vi "Main.vi"(11 "Module Admin":refnum<class "Delacor_lib_QMH_Module Admin.lvclass">) -> ()   [LabVIEW 2019, in "Panther Dashboard.lvlib"]
doc: "Panther Dashboard For DQMH®\n\nDeveloped and maintained by:\nPantherLAB\n\nMain Contributor- Developer:\n\n» Enrique Noé Arias\n\nBrainstorming & Code Reviews:\n\n» Matthias Baudot\n» Fabiola De La Cueva\n» Christopher Farmer\n» Cyril Gambini\n» Joerg Hampel\n» Olivier Jourdan\n» Cesar Muñoz\n» Darren Nattinger\n» Luis Orozco\n» Sam Taggart\n» Diego Torres"
uses:
  Panther Dashboard.lvlib
  <vilib>/Delacor/Delacor QMH/Libraries/Module Admin_class/Delacor_lib_QMH_Module Admin.lvclass
  refresh--button.ctl
  Module Data--cluster.ctl
  Maps List and refs--cluster.ctl
  <vilib>/National Instruments/Tree Map/Tree Map Data.ctl
  DQMH Modules Info--cluster.ctl
  Module type--enum.ctl
  Project References--cluster.ctl
  Selection Type--enum.ctl
  <vilib>/Delacor/Delacor QMH/Libraries/Module Admin_class/Delacor_lib_QMH_Module Admin.lvclass/Delacor_lib_QMH_Module Admin.ctl
  References Updated Argument--cluster.ctl
  DQMH Tools Menu--enum.ctl
  <vilib>/Delacor/Delacor QMH/Libraries/Message Queue_class/Delacor_lib_QMH_Message Queue.lvclass/Delacor_lib_QMH_Message Queue.ctl
  Expand Results Argument--cluster.ctl
  Execute Default Event Request Argument--cluster.ctl
  Tree DQMH Selection Argument--cluster.ctl
  Scan DQMH Modules Argument--cluster.ctl
  Stop Argument--cluster.ctl
  <vilib>/Utility/miscctls.llb/LVPointTypeDef.ctl
  <vilib>/Delacor/Delacor QMH/Libraries/Message Queue_class/Delacor_lib_QMH_Enqueue Message (Single).vi
  <vilib>/Delacor/Delacor QMH/Libraries/Module Admin_class/Delacor_lib_QMH_Get External Launch.vi
  <vilib>/National Instruments/Tree Map/API/List Roots.vi
  <vilib>/National Instruments/Tree Map/Utility/Into Tree Control Items.vi
  <vilib>/Platform/browser.llb/Open URL in Default Browser (string).vi
  <vilib>/Platform/browser.llb/Open URL in Default Browser (path).vi
  <vilib>/Utility/error.llb/Error Cluster From Error Code.vi
  <vilib>/ErrorRing/Error Ring.xnode
  <vilib>/Delacor/Delacor QMH/Libraries/Message Queue_class/Delacor_lib_QMH_Message Queue.lvclass
  <vilib>/National Instruments/Tree Map/Tree Map.lvlib
  <vilib>/Delacor/Delacor QMH/Libraries/Scripting API/DQMH_Scripting API.lvlib
panel:
  in  "Targets":string(combo)
  in  "Projects":string(combo)
  in  "Expanded Results":bool
  in  "Include Dependencies":bool
  in  "Scan Project":T1
  in  "Modules Tree":string(tree) caption="Tree 2"
  in  "Validate Module":bool
  in  "Edit":bool
  in  "Edit":bool
  in  "Module Description":string
  out "Event Connector Pane":picture
  in  "Event Description":string
  in  "Module ID":i32=-1 min=-1 max=1000 step=1 format="Module ID %d"
  in  "Create Module Template":bool
  in  "Create RT Tester":bool
  in  "Add Unit Test":bool
  in  "Rename Module":bool
  in  "Add Module":bool
  in  "Rename Event":bool
  in  "Convert Event":bool
  in  "Remove Event":bool
  in  "Add Event":bool
  out "Progress":u16(slide) scale=0.0..1.0
  out "Messages":string
  in  "Theme":bool=TRUE
  in  "About":bool=TRUE
  out "error out":errorcluster
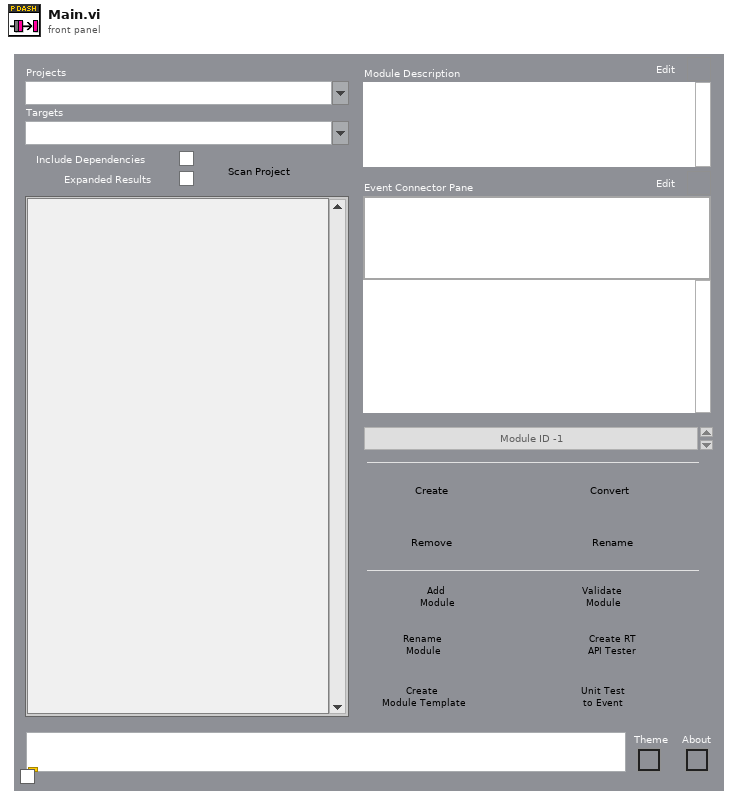
[diagram p1: front panel]
types:
  T1 = typedef "Panther Dashboard.lvlib/refresh--button.ctl" = bool
  T2 = typedef "Panther Dashboard.lvlib/Broadcast Events--cluster.ctl" = cluster{"Module Did Init":refnum<user-event>, "Status Updated":refnum<user-event>, "Error Reported":refnum<user-event>, "Module Did Stop":refnum<user-event>, "Update Module Execution Status":refnum<user-event>, "References Updated":refnum<user-event>, "Projects Updated":refnum<user-event>, "Targets Updated":refnum<user-event>}
  T3 = typedef "Panther Dashboard.lvlib/Request Events--cluster.ctl" = cluster{"Stop Module":refnum<user-event>, "Show Panel":refnum<user-event>, "Hide Panel":refnum<user-event>, "Get Module Execution Status":refnum<user-event>, "Show Diagram":refnum<user-event>, "Scan DQMH Modules":refnum<user-event>, "Tree DQMH Selection":refnum<user-event>, "Open Module API Tester":refnum<user-event>, "Execute Default Event Request":refnum<user-event>, "Expand Results":refnum<user-event>}
  T4 = typedef "Panther Dashboard.lvlib/Selection Type--enum.ctl" = enum16{"Broadcast", "Request", "Module", "Public API"}
  T5 = typedef "Panther Dashboard.lvlib/Module Data--cluster.ctl" = cluster{"Maps":T6, "DQMH Scan Results":T8, "Current Selection":cluster{"VI Ref":refnum<vi>, "DQMH Lib Ref":refnum<vi>}, "Status":string, "Module type":T9, "Module ID":i32, "Theme":bool, "Broadcast?":bool}
  T6 = typedef "Panther Dashboard.lvlib/Maps List and refs--cluster.ctl" = cluster{"Tree Map":T7, "References Map":map{string, refnum<vi>}}
  T7 = typedef "Tree Map.lvlib/Tree Map Data.ctl" = map{string, cluster{"Child Paths Set":set{string}, "Name":string, "Data":string, "Attributes":map{string, string}}}
  T8 = typedef "Panther Dashboard.lvlib/DQMH Modules Info--cluster.ctl" = cluster{"All DQMH Modules Refs":refnum<vi>[], "All Modules Descriptions":string[], "All Modules type":T9[], "Project References":T10}
  T9 = typedef "Panther Dashboard.lvlib/Module type--enum.ctl" = enum16{"Module type: Singleton", "Module type: Cloneable"}
  T10 = typedef "Panther Dashboard.lvlib/Project References--cluster.ctl" = cluster{"Project Ref":refnum<vi>, "Project Name":string, "Target":refnum<vi>, "App Ref":refnum<vi>}
  T11 = typedef "Panther Dashboard.lvlib/References Updated Argument--cluster.ctl" = cluster{"Modules":refnum<vi>[], "Modules Types":T9[], "Application Instance":refnum<vi>}
  T12 = typedef "Panther Dashboard.lvlib/DQMH Tools Menu--enum.ctl" = enum16{"Create New DQMH Event", "Remove DQMH Event", "Convert DQMH Event", "Rename DQMH Event", "Add New DQMH Module", "Create RT Tester", "Rename DQMH Module", "Validate DQMH Module", "Create DQMH Module Template", "New DQMH  Unit Test"}
  T13 = enum8{"Enabled", "Disabled", "Disabled and Grayed Out"}
  T14 = typedef "Panther Dashboard.lvlib/Expand Results Argument--cluster.ctl" = cluster{"Expand?":bool}
  T15 = typedef "Panther Dashboard.lvlib/Execute Default Event Request Argument--cluster.ctl" = cluster{"Event Name":string}
  T16 = typedef "Panther Dashboard.lvlib/Tree DQMH Selection Argument--cluster.ctl" = cluster{"Tree DQMH Sel":string}
  T17 = typedef "Panther Dashboard.lvlib/Scan DQMH Modules Argument--cluster.ctl" = cluster{"Include Dependencies":bool, "Project":string, "Target":string}
  T18 = enum32{"invalid lock state", "Not Locked", "Locked (No Password)", "Password-protected"}
  T19 = typedef "Panther Dashboard.lvlib/Stop Argument--cluster.ctl" = cluster{"Origin":string, "Exit via Stop Module Req?":bool, "Wait for Module to stop?":bool}
  T20 = typedef "LVPointTypeDef.ctl" = cluster{"Horizontal":i16, "Vertical":i16}
  T21 = enum32{"Invalid", "Standard", "Closed", "Hidden", "Minimized", "Maximized"}
  T22 = cluster{"Left Cell String":string, "Child Text":string[], "Child Tag":string, "Item Indent":i32, "Child Only?":bool, "Glyph Index":i32}[]
  T23 = typedef "Panther Dashboard.lvlib/Documentation--cluster.ctl" = cluster{"Module Description":string, "Event Description":string}
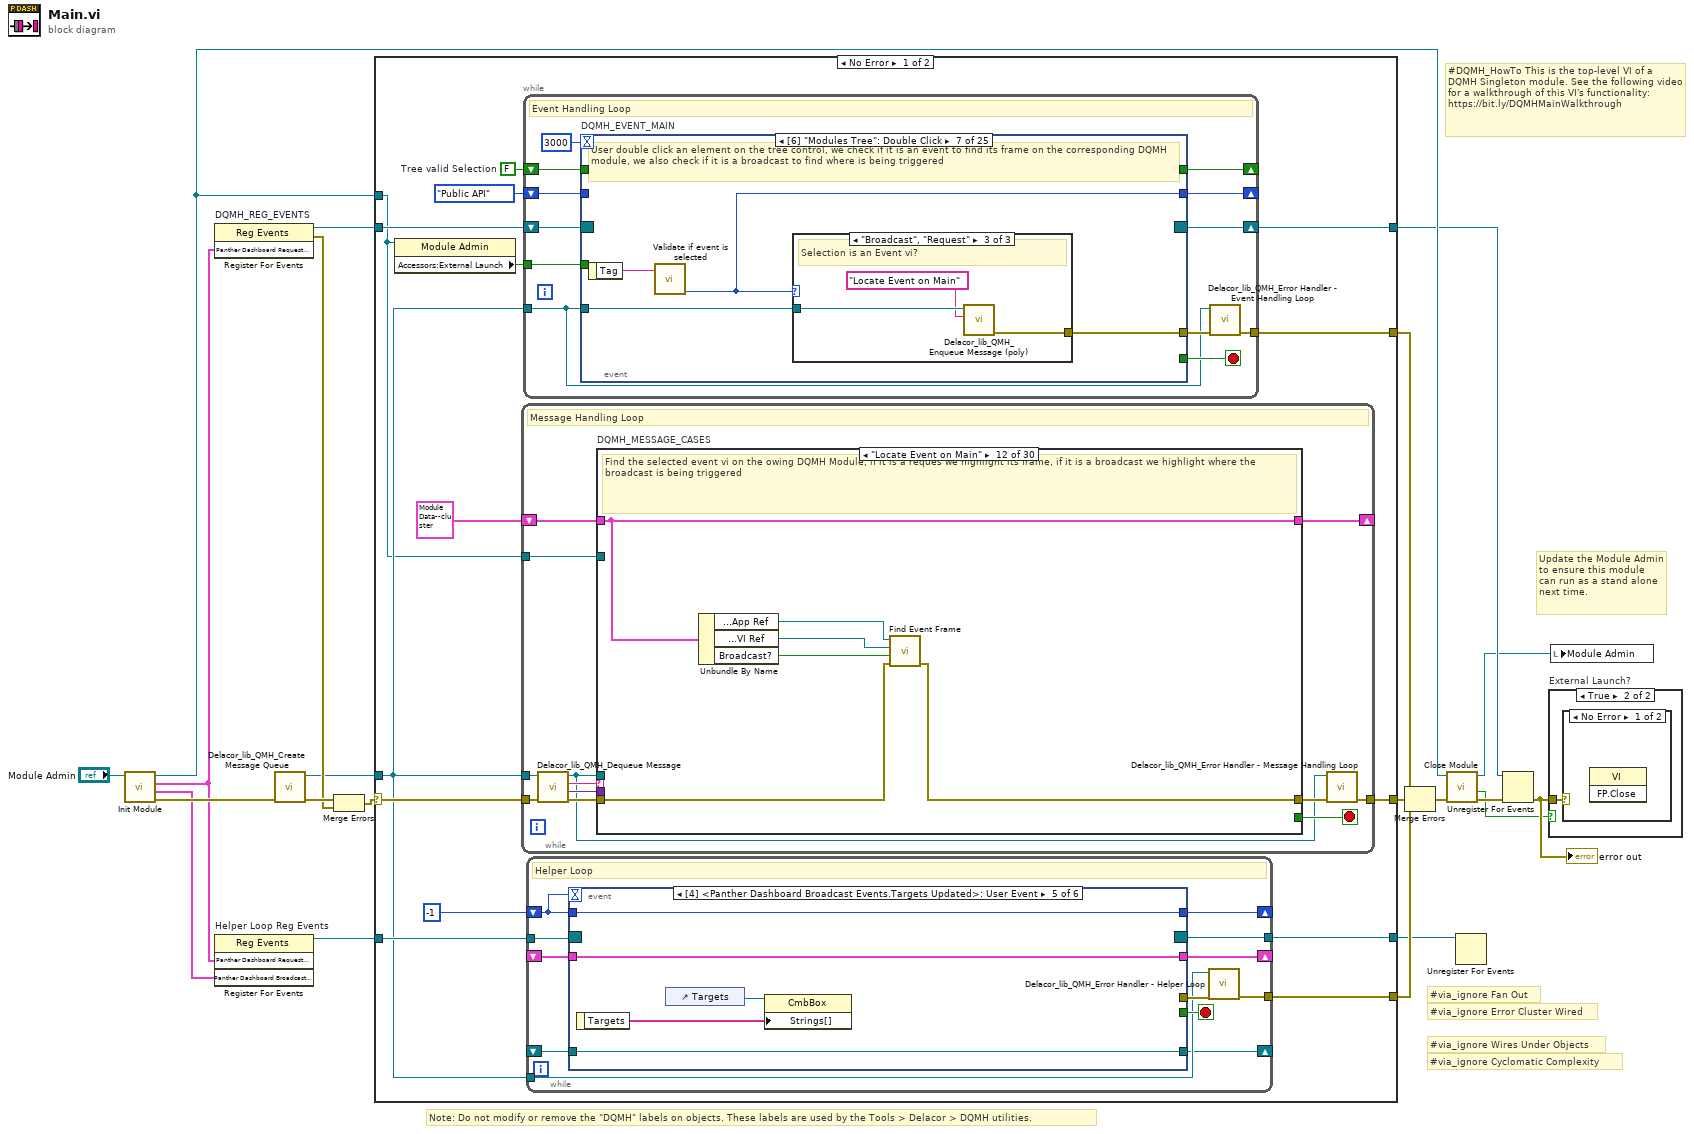
[diagram p0: block diagram]
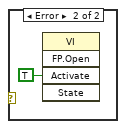
[diagram p3: hidden frame]
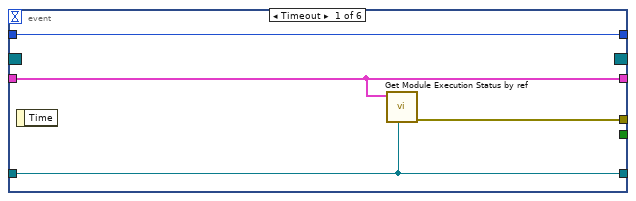
[diagram p4: hidden frame]
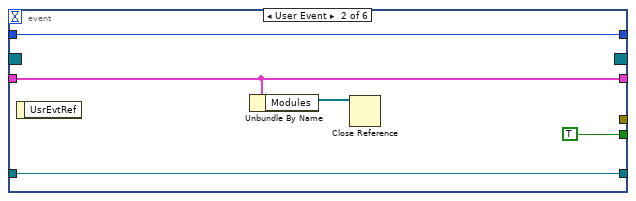
[diagram p5: hidden frame]
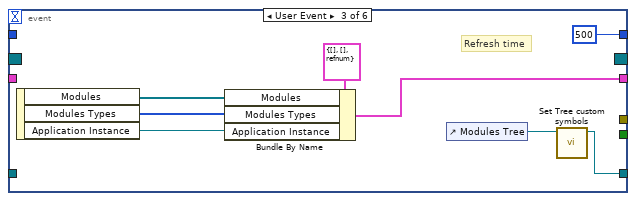
[diagram p6: hidden frame]
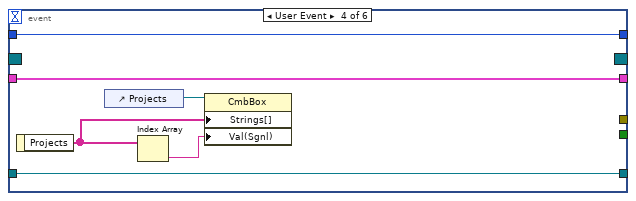
[diagram p7: hidden frame]
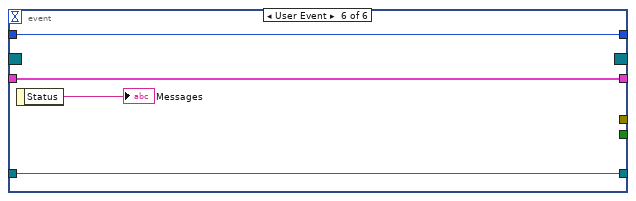
[diagram p8: hidden frame]
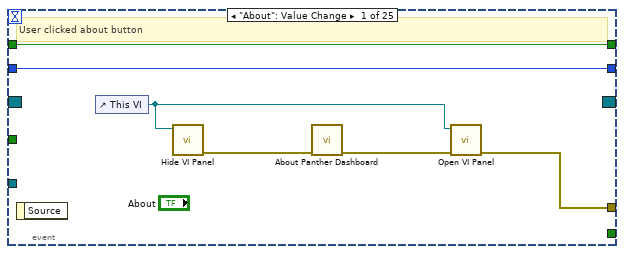
[diagram p9: hidden frame]
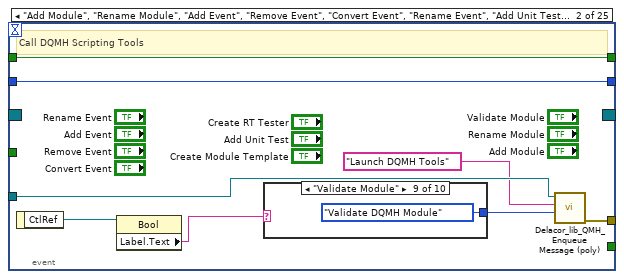
[diagram p10: hidden frame]
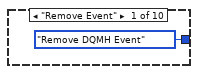
[diagram p11: hidden frame]
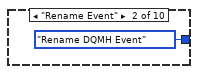
[diagram p12: hidden frame]
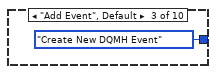
[diagram p13: hidden frame]
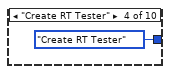
[diagram p14: hidden frame]
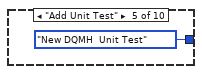
[diagram p15: hidden frame]
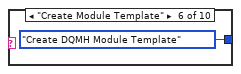
[diagram p16: hidden frame]
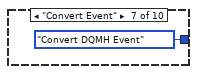
[diagram p17: hidden frame]
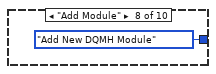
[diagram p18: hidden frame]
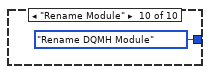
[diagram p19: hidden frame]
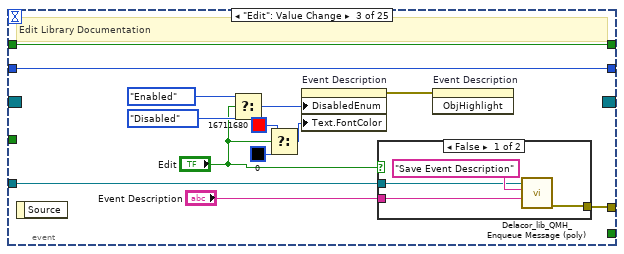
[diagram p20: hidden frame]
diagram:
  # "#via_ignore Fan Out"
  # "#via_ignore Cyclomatic Complexity"
  # "#via_ignore Wires Under Objects"
  # "#via_ignore Error Cluster Wired"
  # "#DQMH_HowTo This is the top-level VI of a DQMH Singleton module. See the following video for a walkthrough of this VI's functionality: https://bit.ly/DQMHMainWalkthrough"
  # "Note: Do not modify or remove the \"DQMH\" labels on objects. These labels are used by the Tools > Delacor > DQMH utilities."
  # "Update the Module Admin to ensure this module can run as a stand alone next time."
  n1 = call "Init Module.vi"("Singleton Module Admin in"="Module Admin") -> ("error out"=w20:errorcluster, "Panther Dashboard Broadcast Events"=w1:T2, "Panther Dashboard Request Events"=w2:T3, "Singleton Module Admin out"=w11:refnum<class "Delacor_lib_QMH_Module Admin.lvclass">)  [unwired: 7 in]
  n2 = register-events "DQMH_REG_EVENTS"(w2) -> (reference out=w9:refnum<event-registration>, error out=w13:errorcluster)  [unwired: 2 in]
  n3 = register-events "Helper Loop Reg Events"(w2, w1) -> (reference out=w4:refnum<event-registration>)  [unwired: 2 in, 1 out]
  n4 = call <vilib>:"Delacor_lib_QMH_Create Message Queue.vi"("error in"=w20) -> ("error out"=w15:errorcluster, "Message Queue"=w8:refnum<class "Delacor_lib_QMH_Message Queue.lvclass">)  [unwired: 9 in]
  n5 = Merge Errors(w15, w13) -> (w14:errorcluster)
  n6 = case shown="No Error" w14 {
    selector: w14 -> [w34 w689]
    tunnel: [w36 w688] -> w21
    tunnel: [w32 w687] -> w10
    tunnel: w9 -> [w30 w687]
    tunnel: w8 -> [w26 w682]
    tunnel: [w35 _] -> w18
    tunnel: w11 -> [w23 w683]
    tunnel: w4 -> [w29 w681]
    tunnel: [w28 w681] -> w3
    tunnel: [w33 _] -> w12
    frame No Error {
      w25 = FALSE  # Tree valid Selection
      n7 = property class="Module Admin"(reference=w23) -> ("Accessors:External Launch"=w22:bool)  [unwired: 1 in, 2 out]
      n8 = while {
        tunnel: w26 -> [w326]
        shift-right: [w330] -> _
        shift-left: T5 {"Maps"={"Tree Map"={}, "References Map"={}}, "DQMH Scan Results"={"All DQMH Modules Refs"=[], "All Modules Descriptions"=[], "All Modules type"=[], "Project References"={"Project Ref"=refnum, "Project Name"="", "Target"=refnum, "App Ref"=refnum}}, "Current Selection"={"VI Ref"=refnum, "DQMH Lib Ref"=refnum}, "Status"="", "Module type"=enum."Module type: Singleton", "Module ID"=0, "Theme"=FALSE, "Broadcast?"=FALSE} ("Data Cluster") -> [w331]
        tunnel: w34 -> [w334]
        tunnel: [w332] -> w36
        tunnel: w23 -> [w324]
        stop <- w329 stop-if-true
        # "Message Handling Loop"
        n9 = call-dynamic "Delacor_lib_QMH_Dequeue Message.vi"("error in"=w334, "Message Queue in"=w326) -> ("error out"=w333:errorcluster, "Message Data"=w327:variant, "Message"=w328:string, "Message Queue out"=w325:refnum<class "Delacor_lib_QMH_Message Queue.lvclass">)  [unwired: 6 in]
        n10 = case "DQMH_MESSAGE_CASES" shown="\"Locate Event on Main\"" w328 {
          selector: w328 -> [_ w379 _ _ _ _ _ _ _ _ _ _ _ _ _ _ w551 _ w574 _ _ _ _ _ _ _ _ _ _ w668]
          tunnel: w325 -> [w346 _ _ _ _ _ _ _ _ _ _ _ _ _ _ _ _ _ _ _ _ _ _ _ _ _ _ w638 w660 _]
          tunnel: w333 -> [w364 w382 w384 w408 w416 w423 w430 w456 w472 w477 w478 w484 w502 w518 w537 w544 w556 w569 w579 w592 w599 w606 w609 w620 w628 w633 w635 w645 w666 w670]
          tunnel: [w363 w375 w384 w407 w415 w423 w430 w455 w471 w476 w483 w489 w500 w516 w539 w543 w554 w570 w577 w584 w598 w605 w608 w620 w624 w632 w635 w641 w663 w671] -> w335
          tunnel: w331 -> [w352 w381 w383 w395 w413 w421 w429 w451 w467 w475 w482 w488 w495 w514 w541 w546 w550 w567 w573 w591 w597 w604 w611 w619 w629 w631 w634 w640 w652 w669]
          tunnel: [w351 w381 w383 w400 w413 w421 w429 w445 w467 w475 w482 w488 w495 w514 w541 w546 w548 w567 w571 w587 w595 w604 w611 w619 w629 w631 w634 w640 w652 w669] -> w330
          tunnel: [_ _ _ _ _ _ _ _ _ _ _ _ _ _ _ _ _ _ _ _ _ _ _ _ _ _ _ _ w659 _] -> w329
          tunnel: w327 -> [_ w380 _ w403 _ _ _ w454 w469 _ _ _ w498 _ _ _ w552 _ w575 w589 w596 w603 _ _ _ _ _ w639 w658 _]
          tunnel: w324 -> [w353 _ _ _ _ _ _ _ _ _ _ _ _ _ _ _ _ _ _ _ _ _ _ _ _ _ _ w637 w653 _]
          frame "Initialize" {
            w343 = "Panther Dashboard for DQMH" ("format string")
            # "#via_ignore Overlapping Controls"
            # "Scripting not\nallowed on RTE"
            # "Initialize - Any operation that needs to be done before the module can receive messages. Synchronize Caller Events.vi will inform Start Module.vi that the module has launched and is ready to receive messages. Module Did Init.vi will broadcast that the module initialized."
            n11 = call "Synchronize Caller Events.vi"("error in (no error)"=w364, "Singleton Module Admin in"=w353) -> ("error out"=w361:errorcluster, "Singleton Module Admin out"=w348:refnum<class "Delacor_lib_QMH_Module Admin.lvclass">)  [unwired: 8 in]
            n12 = invoke on="Modules Tree" class="Tree (strict)" method="Edit Tree Items.Delete"() -> ()  [unwired: 5 in, 5 out]
            n13 = property on="Property Node" class="Module Admin"(reference=w348) -> ("Accessors:External Launch"=w357:bool)  [unwired: 1 in, 2 out]
            n14 = call "Scan For App Projects.vi"("error in"=w361) -> ("error out"=w360:errorcluster)  [unwired: 10 in]
            n15 = Select(t=T21."Hidden" ("State"), s=w357, f=T21."Standard" ("State")) -> (s? t:f=w354:T21)
            n16 = property on="Event Connector Pane" class="Pict"("Origin"=T20 {"Horizontal"=-5, "Vertical"=-3}) -> ()  [unwired: 2 in, 2 out]
            n17 = call "Module Name--constant.vi"() -> ("Module Name"=w349:string)  [unwired: 11 in]
            n18 = property on="Property Node" class="VI"("Front Panel.Title"=w343, "Front Panel.IsFrontmost"=TRUE ("Front Panel Window:Is Frontmost")) -> (reference out=w359:refnum<vi>, error out=w366:errorcluster)  [unwired: 2 in]
            n19 = call "Module Did Init.vi"("error in (no error)"=w360, "Initialized?"=TRUE, "Origin"=w349) -> ("error out"=w338:errorcluster)  [unwired: 8 in]
            n20 = invoke on="Invoke Node" class="VI" method="FP.Open"(reference=w359, error in=w366, "State"=w354) -> (reference out=w358:refnum<vi>, error out=w365:errorcluster)  [unwired: 2 in, 3 out]
            n21 = call "Read Theme from Config.vi"("error in"=w338) -> ("error out"=w337:errorcluster, "Theme"=w336:bool)  [unwired: 9 in]
            n22 = property on="Modules Tree" class="Tree (strict)"("Allow Item Drag"=TRUE ("Drag/Drop:Allow Dragging"), "SelColor"=u32 8355711) -> ()  [unwired: 2 in, 2 out]
            n23 = invoke on="Invoke Node" class="VI" method="FP.Center"(reference=w358, error in=w365) -> (reference out=w344:refnum<vi>, error out=w362:errorcluster)  [unwired: 1 in, 1 out]
            n24 = Bundle By Name(cluster=w352, "Module ID"=-1, "Status"=w343) -> (w351:T5)
            n25 = local write "Messages"(w343) -> ()
            n26 = disable-structure shown="RUN_TIME_ENGINE==True" {
              disable-tunnel: w337 -> [w371 w374]
              disable-tunnel: [w370 w373] -> w363
              disable-tunnel: w346 -> [w369 _]
              disable-tunnel: w336 -> [w367 _]
              frame condition #0 (active) {
                n27 = call-poly <vilib>:"Delacor_lib_QMH_Enqueue Message (poly).vi"("error in"=w371, "Message Data"=w367, "Message"="Theme", "Message Queue in"=w369) -> ("error out"=w370:errorcluster)  [unwired: 6 in, 1 out]
              }
              frame condition #1 {
                n28 = call "Stop Module.vi"("error in"=w374, "Origin"="Self") -> ("error out"=w373:errorcluster)  [unwired: 9 in]
              }
            }
            n29 = invoke class="VI" method="Default Vals.Reinit All"(reference=w344, error in=w362) -> ()  [unwired: 1 in, 3 out]
            "Progress" <- u16 0 ("Progress")
          }
          frame "Refresh Targets" {
            # "When the User selects a Project triggers this task to scan all the targets available"
            n30 = Variant To Data(error in=w382, type=w379, Variant=w380) -> (data=w378:string, error out=w377:errorcluster)
            n31 = call "Get all Targets.vi"("error in"=w377, "Project Selection"=w378) -> ("error out"=w375:errorcluster, "Targets"=w376:string[])  [unwired: 8 in]
            n32 = call "Targets Updated.vi"("Targets"=w376) -> ()  [unwired: 10 in, 1 out]
          }
          frame "---Module Specific---" {
            # "Separator -- The following cases handle messages specific to this Module."
          }
          frame "Scan DQMH Modules" {
            # "Scan DQMH Modules in the project and fill 2 maps one with the Vi References and the another one with the list of DQMH modules on the project"
            n33 = Variant To Data(error in=w408, type=T17 {"Include Dependencies"=FALSE, "Project"="", "Target"=""} ("Scan DQMH Modules Argument"), Variant=w403) -> (data=w401:T17, error out=w386:errorcluster)
            n34 = Unbundle By Name(w401) -> ("Project"=w388:string, "Target"=w390:string, "Include Dependencies"=w391:bool)
            n35 = invoke on="Modules Tree" class="Tree (strict)" method="Edit Tree Items.Delete"(error in=w386) -> ()  [unwired: 4 in, 5 out]
            n36 = call "Close vi references.vi"("Data Cluster"=w395) -> ("error out"=w404:errorcluster)  [unwired: 10 in]
            n37 = disable-structure shown="Disabled" {
              disable-tunnel: w386 -> [w409 _]
              frame Disabled {
                n38 = call <vilib>:"Set Busy.vi"("error in (no error)"=w409) -> ()  [unwired: 9 in, 2 out]
              }
              frame Enabled {
              }
            }
            n39 = local write "Include Dependencies"(w391) -> ()
            n40 = Format Into String(format string="Panther Dashboard for DQMH: %s", w388) -> (resulting string=w392:string)  [unwired: 2 in, 1 out]
            n41 = control-ref of="Progress"() -> (w387:refnum<vi>)
            n42 = local read "Expanded Results"() -> (w394:bool)
            n43 = property on="Property Node" class="VI"("Front Panel.Title"=w392) -> ()  [unwired: 2 in, 2 out]
            n44 = call "Scan DQMH Modules and create Maps.vi"("Progress bar"=w387, "error in"=w404, "Include Dependencies"=w391, "Target Selection"=w390, "Project"=w388) -> ("error out"=w406:errorcluster, "Tree Map out"=w389:T7, "map ref out"=w396:map{string, refnum<vi>}, "DQMH Modules Info"=w399:T8)  [unwired: 3 in]
            n45 = control-ref of="Modules Tree"() -> (w397:refnum<vi>)
            n46 = Bundle By Name(cluster=w395, "DQMH Scan Results"=w399, "Maps.References Map"=w396, "Maps.Tree Map"=w389) -> (w400:T5)
            n47 = call "Expand Results.vi"("error in"=w406, "Expand?"=w394) -> ("error out"=w405:errorcluster)  [unwired: 9 in]
            n48 = call <vilib>:"Tree Map to Tree Control Items.vi"("Tree Map In"=w389) -> ("Tree Control Items"=w398:T22)  [unwired: 10 in]
            n49 = call "Draw Tree.vi"("Tree Control Items"=w398, "TreeControl in"=w397) -> ("error out"=w385:errorcluster)  [unwired: 9 in]
            n50 = Merge Errors(w386, w405) -> (w407:errorcluster)
            n51 = call <vilib>:"Unset Busy.vi"("error in (no error)"=w385) -> ()  [unwired: 10 in, 1 out]
          }
          frame "Drag VI" {
            # "This is the functionality alowing drag and drop the current selection to your code, you can build code using panther Dashboard."
            n52 = Unbundle By Name(w413) -> ("DQMH Scan Results.Project References.App Ref"=w412:refnum<vi>, "DQMH Scan Results.Project References.Target"=w411:refnum<vi>, "Current Selection.VI Ref"=w410:refnum<vi>)
            n53 = call "Drop Event into subVI.vi"("Current Selection.VI Ref"=w410, "Target"=w411, "App Ref"=w412) -> ("error out"=w414:errorcluster)  [unwired: 8 in]
            n54 = Merge Errors(w414, w416) -> (w415:errorcluster)
          }
          frame "Who is launching this module?" {
            w422 = 0  # Start Module.vi index
            # "Find all the VIS calling the Start Module.vi of the selected module library"
            n55 = Unbundle By Name(w421) -> ("Theme"=w420:bool, "DQMH Scan Results.Project References.App Ref"=w419:refnum<vi>, "DQMH Scan Results.Project References.Target"=w418:refnum<vi>, "Current Selection.DQMH Lib Ref"=w417:refnum<vi>)
            n56 = call "Find some Public API VI.vi"("Theme"=w420, "Public Api file index"=w422, "Library in"=w417, "Target"=w418, "App Ref"=w419) -> ()  [unwired: 7 in]
          }
          frame "Who is registered to this module's broadcasts?" {
            w428 = 2  # Obtain Broadcast Events for Registration.vi index
            # "Find all the VIS calling the Obtain broadcast events for registration of the selected module library"
            n57 = Unbundle By Name(w429) -> ("Theme"=w427:bool, "DQMH Scan Results.Project References.App Ref"=w426:refnum<vi>, "DQMH Scan Results.Project References.Target"=w425:refnum<vi>, "Current Selection.DQMH Lib Ref"=w424:refnum<vi>)
            n58 = call "Find some Public API VI.vi"("Theme"=w427, "Public Api file index"=w428, "Library in"=w424, "Target"=w425, "App Ref"=w426) -> ()  [unwired: 7 in]
          }
          frame "Tree DQMH Selection" {
            # "There is a new selection of the DQMH Tree list, need to search and update indicators acordanly."
            n59 = Unbundle By Name(w451) -> ("Maps.Tree Map"=w450:T7, "Maps.References Map"=w449:map{string, refnum<vi>}, "DQMH Scan Results"=w448:T8)
            n60 = Variant To Data(error in=w456, type=T16 {"Tree DQMH Sel"=""} ("Tree DQMH Selection Argument"), Variant=w454) -> (data=w452:T16, error out=w455:errorcluster)
            n61 = Unbundle By Name(w452) -> ("Tree DQMH Sel"=w442:string)
            n62 = call "Get List Information.vi"("List Selection"=w442, "DQMH Scan Info"=w448, "References Map"=w449, "Tree Map"=w450) -> ("Documentation"=w446:T23, "Clone?"=w441:bool, "Vi out"=w443:refnum<vi>, "Module type"=w440:T9, "VI Connector Pane"=→"Event Connector Pane":picture, "DQMH Lib"=w444:refnum<vi>, "Broadcast?"=w431:bool)  [unwired: 1 in]
            n63 = Unbundle By Name(w446) -> ("Module Description"=w439:string, "Event Description"=w438:string)
            n64 = control-ref of="Module Description"() -> (w437:refnum<vi>)
            n65 = control-ref of="Event Description"() -> (w436:refnum<vi>)
            n66 = control-ref of="Module ID"() -> (w432:refnum<vi>)
            n67 = Bundle By Name(cluster=w451, "Current Selection.DQMH Lib Ref"=w444, "Current Selection.VI Ref"=w443, "Module type"=w440, "Broadcast?"=w431) -> (w445:T5)
            n68 = Build Array(w439, w438) -> (w434:string[])
            n69 = Build Array(w437, w436) -> (w435:refnum<vi>[])
            n70 = call "Enable disable control.vi"("Enabled?"=w441, "Digital in"=w432) -> ()  [unwired: 10 in]
            n71 = for {
              tunnel: w435 -> [w459] mode=indexing
              tunnel: w434 -> [w458] mode=indexing
              tunnel: bool[] [FALSE, TRUE] ("Adjust Height?") -> [w457] mode=indexing
              n72 = call "Format to Bold.vi"("Adjust Height?"=w457, "String Value"=w458, "String Ref"=w459) -> ()  [unwired: 9 in]
            }
          }
          frame "Launch DQMH Tools" {
            # "Launch DQMH Tools"
            n73 = Variant To Data(error in=w472, type=DQMH_Tools_Menu--enum."Create New DQMH Event" ("DQMH Tools"), Variant=w469) -> (data=w463:T12, error out=w470:errorcluster)
            n74 = Unbundle By Name(w467) -> ("DQMH Scan Results.Project References.Project Name"=w465:string, "DQMH Scan Results.Project References.App Ref"=w466:refnum<vi>, "Current Selection.DQMH Lib Ref"=w461:refnum<vi>)
            n75 = Format Into String(format string="DQMH Tool: %s being executed ", w463) -> (resulting string=w464:string)  [unwired: 2 in, 1 out]
            n76 = call "Status Updated.vi"("Status"=w464) -> ()  [unwired: 10 in, 1 out]
            n77 = property class="Library"(reference=w461) -> ("Name"=w460:string)  [unwired: 1 in, 2 out]
            n78 = call "Launch DQMH Tools by menu.vi"("Project"=w465, "Application Instance"=w466, "error in"=w470, "Module Name"=w460, "DQMH Tools"=w463) -> ("error out"=w471:errorcluster)  [unwired: 6 in]
          }
          frame "Open Module API Tester" {
            # "Open the API Tester from the current DQMH Module Selected"
            n79 = Unbundle By Name(w475) -> ("DQMH Scan Results.Project References.App Ref"=w473:refnum<vi>, "Current Selection.DQMH Lib Ref"=w474:refnum<vi>)
            n80 = call "Open API Tester.vi"("error in"=w477, "DQMH Library Ref"=w474, "Application Instance"=w473) -> ("error out"=w476:errorcluster)  [unwired: 8 in]
          }
          frame "Find Module in project" {
            # "Find the selected module in project explorer"
            n81 = Unbundle By Name(w482) -> ("Current Selection.DQMH Lib Ref"=w481:refnum<vi>, "DQMH Scan Results.Project References.Project Ref"=w480:refnum<vi>, "DQMH Scan Results.All DQMH Modules Refs"=w479:refnum<vi>[])
            n82 = call "Find Library in Project.vi"("error in (no error)"=w478, "DQMH Modules Refs"=w479, "Project Ref"=w480, "DQMH Lib Ref"=w481) -> ("error out"=w483:errorcluster)  [unwired: 7 in]
          }
          frame "Locate Event on Main" {
            # "Find the selected event vi on the owing DQMH Module, if it is a reques we highlight its frame, if it is a broadcast we highlight where the broadcast is being triggered"
            n83 = Unbundle By Name(w488) -> ("DQMH Scan Results.Project References.App Ref"=w486:refnum<vi>, "Current Selection.VI Ref"=w487:refnum<vi>, "Broadcast?"=w485:bool)
            n84 = call "Find Event Frame.vi"("error in"=w484, "Broadcast?"=w485, "VI in"=w487, "Application Instance"=w486) -> ("error out"=w489:errorcluster)  [unwired: 7 in]
          }
          frame "Execute Default Event Request" {
            # "Execute Default Event"
            n85 = Variant To Data(error in=w502, type=T15 {"Event Name"=""} ("Execute Default Event Request Argument"), Variant=w498) -> (data=w496:T15, error out=w501:errorcluster)
            n86 = Unbundle By Name(w495) -> ("DQMH Scan Results.Project References.App Ref"=w494:refnum<vi>, "Current Selection.DQMH Lib Ref"=w493:refnum<vi>, "Module ID"=w491:i32, "Module type"=w490:T9)
            n87 = Unbundle By Name(w496) -> ("Event Name"=w492:string)
            n88 = call "Execute Default event.vi"("Module type"=w490, "Module ID"=w491, "Event"=w492, "DQMH Library Ref"=w493, "application Instance"=w494) -> ("error out"=w499:errorcluster)  [unwired: 6 in]
            n89 = Merge Errors(w501, w499) -> (w500:errorcluster)
          }
          frame "Search for Event Callers / listeners" {
            # "Invalid Ref"
            # "Search for this event callers"
            n90 = Unbundle By Name(w514) -> ("Broadcast?"=w506:bool, "Theme"=w512:bool, "DQMH Scan Results.Project References.Project Ref"=w504:refnum<vi>, "Current Selection.VI Ref"=w511:refnum<vi>)
            n91 = Select(t="Searching code registered to current broadcast selection" ("Status"), s=w506, f="Searching for Event Callers" ("Status")) -> (s? t:f=w507:string)
            n92 = call "Status Updated.vi"("error in (no error)"=w518, "Status"=w507) -> ("error out"=w517:errorcluster)  [unwired: 9 in]
            n93 = case shown="False" w506 {
              tunnel: w517 -> [w523 w530]
              tunnel: [w522 w529] -> w503
              tunnel: w511 -> [w521 w526]
              tunnel: [w520 w528] -> w510
              tunnel: w504 -> [w519 w527]
              frame False {
                # "Requests"
                n94 = call <vilib>:"Get Callers of Request VI in Project.vi"("error in"=w523, "Request VI"=w521, "Project"=w519) -> ("error out"=w522:errorcluster, "Request VI Callers"=w520:refnum<vi>[])  [unwired: 7 in]
              }
              frame True {
                # "Broadcast"
                n95 = Two Button Dialog(message="This is an exhaustive task that can take up to minutes, do you wish to continue?") -> (T button?=w525:bool)  [unwired: 2 in]
                n96 = case shown="True" w525 {
                  tunnel: w530 -> [w531 w536]
                  tunnel: [w531 w535] -> w529
                  tunnel: [_ w534] -> w528
                  tunnel: w527 -> [_ w533]
                  tunnel: w526 -> [_ w532]
                  frame False {
                  }
                  frame True {
                    n97 = call <vilib>:"Get VIs Registered for Broadcast in Project.vi"("error in"=w536, "Broadcast VI"=w532, "Project"=w533) -> ("error out"=w535:errorcluster, "VIs Registered for Broadcast"=w534:refnum<vi>[])  [unwired: 7 in]
                  }
                }
              }
            }
            n98 = call <vilib>:"Set Busy.vi"("error in (no error)"=w517) -> ()  [unwired: 9 in, 2 out]
            n99 = call <vilib>:"Clear Errors.vi"("error in (no error)"=w503, "specific error code to clear (0: all)"=5000) -> ("error out"=w515:errorcluster)  [unwired: 4 in, 1 out]
            n100 = call <vilib>:"Unset Busy.vi"("error in (no error)"=w503) -> ()  [unwired: 10 in, 1 out]
            n101 = call "Start Call to results window.vi"("Find Broadcast?"=w506, "Request VI Callers"=w510, "Event"=w511, "Theme"=w512) -> ()  [unwired: 8 in]
            n102 = call <vilib>:"Clear Errors.vi"("error in (no error)"=w515, "specific error code to clear (0: all)"=1026) -> ("error out"=w516:errorcluster)  [unwired: 4 in, 1 out]
          }
          frame "Open VI on Disk" {
            # "Open current event selection on the file system"
            n103 = Unbundle By Name(w541) -> ("Current Selection.VI Ref"=w540:refnum<vi>)
            n104 = property class="VI"(reference=w540) -> ("Path"=w538:path)  [unwired: 1 in, 2 out]
            n105 = call "Open File on Disk.vi"("error in"=w537, "file or directory path"=w538) -> ("error out"=w539:errorcluster)  [unwired: 9 in]
          }
          frame "Open File Library on Disk" {
            # "Open current Module Library selection on the file system"
            n106 = Unbundle By Name(w546) -> ("Current Selection.DQMH Lib Ref"=w545:refnum<vi>)
            n107 = property class="Library"(reference=w545) -> ("Path"=w542:path)  [unwired: 1 in, 2 out]
            n108 = call "Open File on Disk.vi"("error in"=w544, "file or directory path"=w542) -> ("error out"=w543:errorcluster)  [unwired: 9 in]
          }
          frame "Save Library Documentation" {
            # "Save the Library documentation"
            n109 = Variant To Data(error in=w556, type=w551, Variant=w552) -> (data=w549:string, error out=w555:errorcluster)
            n110 = in-place {
              in-place-border: w549 -> [w561]
              in-place-border: [w563] -> w553
              n111 = in-place-cluster #1(w550) -> ("Current Selection.DQMH Lib Ref"=w562:refnum<vi>, "DQMH Scan Results"=w559:T8)
              n112 = call "Save Library Documentation.vi"("New Description"=w561, "DQMH Modules Info In"=w559, "Library in"=w562) -> ("error out"=w563:errorcluster, "DQMH Modules Info Out"=w560:T8, "Lib out"=w558:refnum<vi>)  [unwired: 6 in]
              n113 = property class="Library"(reference=w558) -> ("Description"=w557:string)  [unwired: 1 in, 2 out]
              n114 = local write "Module Description"(w557) -> ()
              n115 = in-place-cluster #1("Current Selection.DQMH Lib Ref"=w558, "DQMH Scan Results"=w560) -> (w548:T5)
            }
            n116 = property on="Module Description" class="Str"("Text.FontColor"=u32 0) -> ()  [unwired: 2 in, 2 out]
            n117 = Merge Errors(w555, w553) -> (w554:errorcluster)
          }
          frame "Edit library Documentation" {
            # "Edit Library Documentation"
            n118 = Unbundle By Name(w567) -> ("Current Selection.DQMH Lib Ref"=w566:refnum<vi>)
            n119 = call "Get library description.vi"("Library in"=w566) -> ("error out"=w568:errorcluster, "Description"=w565:string)  [unwired: 9 in]
            n120 = local write "Module Description"(w565) -> ()
            n121 = property on="Module Description" class="Str"("Text.FontColor"=u32 16711680) -> ()  [unwired: 2 in, 2 out]
            n122 = Merge Errors(w569, w568) -> (w570:errorcluster)
          }
          frame "Save Event Description" {
            # "Save Event Description"
            n123 = Variant To Data(error in=w579, type=w574, Variant=w575) -> (data=w572:string, error out=w578:errorcluster)
            n124 = in-place {
              in-place-border: w572 -> [w582]
              in-place-border: [w583] -> w576
              n125 = in-place-cluster #2(w573) -> ("Current Selection.VI Ref"=w581:refnum<vi>)
              n126 = call "Save Event Description.vi"("Event Description"=w582, "Event Ref in"=w581) -> ("error out"=w583:errorcluster, "Event Ref out"=w580:refnum<vi>)  [unwired: 8 in]
              n127 = in-place-cluster #2("Current Selection.VI Ref"=w580) -> (w571:T5)
            }
            n128 = Merge Errors(w578, w576) -> (w577:errorcluster)
          }
          frame "Theme" {
            # "Switch to Dark or light Theme modue"
            n129 = Variant To Data(error in=w592, type=TRUE, Variant=w589) -> (data=w586:bool, error out=w585:errorcluster)
            n130 = control-ref of="This VI"() -> (w590:refnum<vi>)
            n131 = Bundle By Name(cluster=w591, "Theme"=w586) -> (w587:T5)
            n132 = call "Set Theme.vi"("Dark?"=w586, "VI in"=w590) -> ()  [unwired: 10 in]
            n133 = call "Save Theme in config.vi"("error in"=w585, "Theme"=w586) -> ("error out"=w584:errorcluster)  [unwired: 9 in]
          }
          frame "Module ID Update" {
            # "Module ID Control has value change"
            n134 = Variant To Data(error in=w599, type=0 ("Module ID"), Variant=w596) -> (data=w594:i32, error out=w598:errorcluster)
            n135 = Bundle By Name(cluster=w597, "Module ID"=w594) -> (w595:T5)
          }
          frame "Expand or Close" {
            # "Expand or Close DQMH Tree control"
            n136 = Variant To Data(error in=w606, type=T14 {"Expand?"=FALSE} ("Expand or Close Argument"), Variant=w603) -> (data=w601:T14, error out=w605:errorcluster)
            n137 = Unbundle By Name(w601) -> ("Expand?"=w600:bool)
            n138 = invoke on="Modules Tree" class="Tree (strict)" method="Open/Close.Open/Close All"("Open"=w600) -> ()  [unwired: 3 in, 4 out]
          }
          frame "Open Project Folder" {
            n139 = Unbundle By Name(w611) -> ("DQMH Scan Results.Project References.Project Ref"=w610:refnum<vi>)
            n140 = property class="Project"(reference=w610) -> ("Path"=w607:path)  [unwired: 1 in, 2 out]
            n141 = call <vilib>:"Show in File System.vi"("error in (no error)"=w609, "file or directory path"=w607) -> ("error out"=w608:errorcluster)  [unwired: 9 in]
          }
          frame "Open Antidoc Output" {
            # "When there is antidoc output"
            n142 = Unbundle By Name(w619) -> ("DQMH Scan Results.Project References.Project Ref"=w618:refnum<vi>)
            n143 = property class="Project"(reference=w618) -> ("Path"=w617:path)  [unwired: 1 in, 2 out]
            n144 = Strip Path(path=w617) -> (stripped path=w616:path)  [unwired: 1 out]
            n145 = Build Path(base path=w616, name or relative path=path "Antidoc-Output/Project-Documentation.adoc") -> (appended path=w615:path)
            n146 = call <vilib>:"Check if File or Folder Exists.vi"("path"=w615) -> ("file or folder exists?"=w613:bool, "dup path"=w614:path)  [unwired: 8 in, 1 out]
            n147 = case shown="False" w613 {
              tunnel: w614 -> [_ w623]
              frame False {
                n148 = call "Status Updated.vi"("Status"="No Antidoc Output has been found") -> ()  [unwired: 10 in, 1 out]
                n149 = call-poly <vilib>:"Open URL in Default Browser.vi"("URL"="https://www.vipm.io/package/wovalab_lib_antidoc/?utm_source=vipm_desktop") -> ()  [unwired: 5 in, 2 out]
              }
              frame True {
                n150 = call-poly <vilib>:"Open URL in Default Browser.vi"("path"=w623) -> ()  [unwired: 5 in, 2 out]
              }
            }
          }
          frame "Edit Project Description" {
            n151 = Unbundle By Name(w629) -> ("DQMH Scan Results.Project References.Project Ref"=w630:refnum<vi>, "Theme"=w627:bool)
            n152 = call "Hide Panel.vi"("error in (no error)"=w628) -> ("error out"=w626:errorcluster)  [unwired: 10 in]
            n153 = call "Project documentation.vi"("error in"=w626, "Theme"=w627, "Project in"=w630) -> ("error out"=w625:errorcluster)  [unwired: 8 in]
            n154 = call "Show Panel.vi"("error in (no error)"=w625) -> ("error out"=w624:errorcluster)  [unwired: 10 in]
          }
          frame "---Copy This Frame---" {
            # "Duplicate this frame when creating new messages.  Change this comment in the duplicated frame to describe this message."
            n155 = Merge Errors(w633) -> (w632:errorcluster)
          }
          frame "---Exit and Error Handling---" {
            # "Separator - The following cases handle errors and exit messages."
          }
          frame "Error" {
            # "Error - Check the error message data and respond accordingly. This message is sent by the \"Error Handler\" VIs at the end of each loop in this application."
            n156 = property on="Property Node" class="Module Admin"(reference=w637) -> ("Accessors:External Launch"=w636:bool)  [unwired: 1 in, 2 out]
            n157 = Variant To Data(error in=w645, type=errorcluster {"status"=FALSE, "code"=0, "source"=""} ("error constant"), Variant=w639) -> (data=w646:errorcluster, error out=w643:errorcluster)
            n158 = call "Error Reported.vi"("Error"=w646) -> ()  [unwired: 10 in, 1 out]
            n159 = case shown="True" w636 {
              tunnel: [w651 _] -> w642
              tunnel: w638 -> [w649 _]
              tunnel: w646 -> [w650 _]
              frame False {
                # "If the module is running standalone, then pop up an error dialog and call the \"Exit\" message."
                n160 = call <vilib>:"Simple Error Handler.vi"("error in (no error)"=w650) -> ()  [unwired: 4 in, 5 out]
                n161 = call-poly <vilib>:"Delacor_lib_QMH_Enqueue Message (poly).vi"("Priority Message? (F)"=TRUE, "Message"="Exit", "Message Queue in"=w649) -> ("error out"=w651:errorcluster)  [unwired: 7 in, 1 out]
              }
              frame True {
                # "If the module was launched externally, calling the Error Reported broadcast VI is the only action performed by the \"Error\" message. The module's caller can then process the error appropriately."
              }
            }
            n162 = Merge Errors(w643, w642) -> (w641:errorcluster)
            n163 = local write "error out"(w641) -> ()
          }
          frame "Exit" {
            w657 = 91  # 91: not all Exit messages will have an argument
            w659 = TRUE  # Stop the VI
            # "Release the message queue reference"
            # "Exit - Exit the application."
            n164 = Variant To Data(error in=w666, type=T19 {"Origin"="", "Exit via Stop Module Req?"=FALSE, "Wait for Module to stop?"=FALSE} ("Stop Argument"), Variant=w658) -> (data=w655:T19, error out=w662:errorcluster)
            n165 = call <vilib>:"Clear Errors.vi"("error in (no error)"=w662, "specific error code to clear (0: all)"=w657) -> ("error out"=w665:errorcluster)  [unwired: 4 in, 1 out]
            n166 = control-ref of="This VI"() -> (w654:refnum<vi>)
            n167 = invoke on="Modules Tree" class="Tree (strict)" method="Edit Tree Items.Delete"() -> ()  [unwired: 5 in, 5 out]
            n168 = call-dynamic "Delacor_lib_QMH_Release Message Queue.vi"("error in"=w665, "Message Queue"=w660) -> ("error out"=w664:errorcluster)  [unwired: 9 in]
            n169 = call "Handle Exit.vi"("Stop Argument"=w655, "Admin in"=w653, "VI reference"=w654) -> ("error out"=w661:errorcluster)  [unwired: 7 in, 1 out]
            n170 = call "Close vi references.vi"("Data Cluster"=w652) -> ()  [unwired: 10 in, 1 out]
            n171 = Merge Errors(w664, w661) -> (w663:errorcluster)
          }
          frame Default {
            # "'Default' case only runs if there is a message that isn't defined in any of the other cases.  Output a programming error."
            n172 = call "Module Name--constant.vi"() -> ("Module Name"=w667:string)  [unwired: 11 in]
            n173 = xnode ("Error Ring")("parameter 0"=w668, "parameter 1"=w667) -> ("error out"=w672:errorcluster)
            n174 = Merge Errors(w670, w672) -> (w671:errorcluster)
          }
        }
        n175 = call-dynamic "Delacor_lib_QMH_Error Handler - Message Handling Loop.vi"("error in"=w335, "Message Queue in"=w325) -> ("dup error in"=w332:errorcluster)  [unwired: 8 in, 1 out]
      }
      n176 = while {
        tunnel: w26 -> [w87]
        shift-right: [w89] -> w32
        shift-left: w30 -> [w90]
        tunnel: [w91] -> w35
        shift-right: [w85] -> _
        shift-left: w25 -> [w84]
        shift-right: [w83] -> _
        shift-left: Selection_Type--enum."Public API" ("Selection type") -> [w82]
        tunnel: w22 -> [w81]
        stop <- w88 stop-if-true
        # "Event Handling Loop"
        n177 = event "DQMH_EVENT_MAIN" shown="[6] \"Modules Tree\": Double Click" {
          selector: w90 -> [_ _ _ _ _ _ _ _ _ _ _ _ _ _ _ _ _ _ _ _ _ _ _ _ _]
          dyn-events: [_ _ _ _ _ _ _ _ _ _ _ _ _ _ _ _ _ _ _ _ _ _ _ _ _] -> w89
          timeout: 3000 -> [_ _ _ _ _ _ _ _ _ _ _ _ _ _ _ _ _ _ _ _ _ _ _ _ _]
          tunnel: [_ _ _ _ _ _ _ _ _ _ _ _ _ _ _ _ _ _ _ _ _ _ TRUE ("Discard?") _ _] -> w88
          tunnel: w87 -> [_ w105 w123 w140 w153 w159 w164 w176 w181 w206 _ w215 _ w229 w237 w245 _ _ w262 w271 _ _ w309 w318 _]
          tunnel: [w93 w106 w129 w146 w154 w160 w165 w177 w182 w207 w212 w216 w219 w230 w238 w246 w250 _ w263 w272 _ _ w312 w320 w323] -> w92
          tunnel: [w98 w100 w118 w139 w148 w156 w162 w173 w179 w202 w208 w218 w227 w232 w234 w240 w248 w252 w256 w269 w284 w297 w301 w315 w322] -> w85
          tunnel: w84 -> [w98 w100 w118 w139 w148 w156 w162 w173 w179 _ w208 w218 w227 w232 w234 w240 w248 w252 w256 w269 w284 w297 w301 w315 w322]
          tunnel: [w97 w99 w117 w134 w147 w155 w161 w172 w178 w200 w210 w217 w226 w231 w233 w239 w247 w251 w255 w268 w283 w296 w300 w314 w321] -> w83
          tunnel: w82 -> [w97 w99 w117 w134 w147 w155 _ w172 w178 _ w210 w217 w226 w231 w233 w239 w247 w251 w255 w268 w283 w296 w300 w314 w321]
          tunnel: w81 -> [_ _ _ _ _ _ _ _ _ _ _ _ _ _ _ _ _ _ _ _ w282 w295 _ _ _]
          event "About": Value Change {
            # "User clicked about button"
            n178 = event-data() -> ()  [unwired: 1 in, 1 out]
            n179 = control-ref of="This VI"() -> (w94:refnum<vi>)
            n180 = call "Hide VI Panel.vi"("VI"=w94) -> ("error out"=w96:errorcluster)  [unwired: 10 in]
            n181 = call "About Panther Dashboard.vi"("error in"=w96) -> ("error out"=w95:errorcluster)  [unwired: 10 in]
            n182 = call "Open VI Panel.vi"("error in (no error)"=w95, "VI"=w94) -> ("error out"=w93:errorcluster)  [unwired: 9 in]
          }
          event "Add Module", "Rename Module", "Add Event", "Remove Event", "Convert Event", "Rename Event", "Add Unit Test", "Create RT Tester", "Create Module Template", "Validate Module": Value Change {
            # "Call DQMH Scripting Tools"
            n183 = event-data() -> ("CtlRef"=w102:refnum<vi>)  [unwired: 1 in]
            n184 = property on="Property Node" class="Bool"(reference=w102) -> ("Label.Text"=w101:string)  [unwired: 1 in, 2 out]
            n185 = case shown="\"Validate Module\"" w101 {
              tunnel: [DQMH_Tools_Menu--enum."Remove DQMH Event" ("DQMH Tools") DQMH_Tools_Menu--enum."Rename DQMH Event" ("DQMH Tools") DQMH_Tools_Menu--enum."Create New DQMH Event" ("DQMH Tools") DQMH_Tools_Menu--enum."Create RT Tester" ("DQMH Tools") DQMH_Tools_Menu--enum."New DQMH  Unit Test" ("DQMH Tools") DQMH_Tools_Menu--enum."Create DQMH Module Template" ("DQMH Tools") DQMH_Tools_Menu--enum."Convert DQMH Event" ("DQMH Tools") DQMH_Tools_Menu--enum."Add New DQMH Module" ("DQMH Tools") DQMH_Tools_Menu--enum."Validate DQMH Module" ("DQMH Tools") DQMH_Tools_Menu--enum."Rename DQMH Module" ("DQMH Tools")] -> w103
              frame "Remove Event" {
              }
              frame "Rename Event" {
              }
              frame "Add Event", Default {
              }
              frame "Create RT Tester" {
              }
              frame "Add Unit Test" {
              }
              frame "Create Module Template" {
              }
              frame "Convert Event" {
              }
              frame "Add Module" {
              }
              frame "Validate Module" {
              }
              frame "Rename Module" {
              }
            }
            n186 = call-poly <vilib>:"Delacor_lib_QMH_Enqueue Message (poly).vi"("Message Data"=w103, "Message"="Launch DQMH Tools", "Message Queue in"=w105) -> ("error out"=w106:errorcluster)  [unwired: 7 in, 1 out]
          }
          event "Edit": Value Change {
            # "Edit Library Documentation"
            n187 = event-data() -> ()  [unwired: 1 in, 1 out]
            n188 = Select(t=T13."Enabled" ("Disabled"), s="Edit", f=T13."Disabled") -> (s? t:f=w125:T13)
            n189 = Select(t=u32 16711680, s="Edit", f=u32 0) -> (s? t:f=w120:u32)
            n190 = property on="Event Description" class="Str"("DisabledEnum"=w125, "Text.FontColor"=w120) -> (error out=w128:errorcluster)  [unwired: 2 in, 1 out]
            n191 = case shown="False" "Edit" {
              tunnel: "Event Description" -> [w132 _]
              tunnel: w123 -> [w130 _]
              tunnel: [w133 _] -> w129
              frame False {
                n192 = call-poly <vilib>:"Delacor_lib_QMH_Enqueue Message (poly).vi"("Message Data"=w132, "Message"="Save Event Description", "Message Queue in"=w130) -> ("error out"=w133:errorcluster)  [unwired: 7 in, 1 out]
              }
              frame True {
              }
            }
            n193 = invoke on="Event Description" class="Str" method="ObjHighlight"(error in=w128) -> ()  [unwired: 2 in, 3 out]
          }
          event "Edit": Value Change {
            # "#via_ignore Duplicate Control Labels"
            # "Edit Library Documentation"
            n194 = event-data() -> ()  [unwired: 1 in, 1 out]
            n195 = Select(t=T13."Enabled" ("Disabled"), s="Edit", f=T13."Disabled") -> (s? t:f=w143:T13)
            n196 = property on="Module Description" class="Str"("DisabledEnum"=w143) -> (error out=w145:errorcluster)  [unwired: 2 in, 1 out]
            n197 = invoke on="Module Description" class="Str" method="ObjHighlight"(error in=w145) -> ()  [unwired: 2 in, 3 out]
            n198 = Select(t="Edit library Documentation", s="Edit", f="Save Library Documentation") -> (s? t:f=w136:string)
            n199 = call-poly <vilib>:"Delacor_lib_QMH_Enqueue Message (poly).vi"("Message Data"="Module Description", "Message"=w136, "Message Queue in"=w140) -> ("error out"=w146:errorcluster)  [unwired: 7 in, 1 out]
          }
          event "Expanded Results": Value Change {
            # "Another Module called the \"Expand or Close\" API Method."
            n200 = event-data() -> ()  [unwired: 1 in, 1 out]
            n201 = Bundle(cluster=T14 {"Expand?"=FALSE} ("Expand or Close Argument"), "Expand?"="Expanded Results") -> (w150:T14)
            n202 = call-poly <vilib>:"Delacor_lib_QMH_Enqueue Message (poly).vi"("Message Data"=w150, "Message"="Expand or Close", "Message Queue in"=w153) -> ("error out"=w154:errorcluster)  [unwired: 7 in, 1 out]
          }
          event "Module ID": Value Change {
            # "#via_ignore Unwired Event Nodes"
            # "Module ID has value change"
            n203 = event-data() -> ()  [unwired: 1 in, 1 out]
            n204 = call-poly <vilib>:"Delacor_lib_QMH_Enqueue Message (poly).vi"("Message Data"="Module ID", "Message"="Module ID Update", "Message Queue in"=w159) -> ("error out"=w160:errorcluster)  [unwired: 7 in, 1 out]
          }
          event "Modules Tree": Double Click {
            # "User double click an element on the tree control, we check if it is an event to find its frame on the corresponding DQMH module, we also check if it is a broadcast to find where is being triggered"
            n205 = event-data() -> ("Tag"=w163:string)  [unwired: 1 in]
            n206 = call "Validate if event is selected.vi"("Tree Selection"=w163) -> ("Selection type"=w161:T4)  [unwired: 10 in]
            n207 = case shown="\"Broadcast\", \"Request\"" w161 {
              tunnel: [w168 _ w171] -> w165
              tunnel: w164 -> [w167 _ w170]
              frame "Module" {
                # "Selection is a module"
                n208 = call-poly <vilib>:"Delacor_lib_QMH_Enqueue Message (poly).vi"("Message"="Find Module in project", "Message Queue in"=w167) -> ("error out"=w168:errorcluster)  [unwired: 8 in, 1 out]
              }
              frame "Public API" {
              }
              frame "Broadcast", "Request" {
                # "Selection is an Event vi?"
                n209 = call-poly <vilib>:"Delacor_lib_QMH_Enqueue Message (poly).vi"("Message"="Locate Event on Main", "Message Queue in"=w170) -> ("error out"=w171:errorcluster)  [unwired: 8 in, 1 out]
              }
            }
          }
          event "Modules Tree": Drag Starting? {
            n210 = event-data() -> ()  [unwired: 1 in, 1 out]
            n211 = call-poly <vilib>:"Delacor_lib_QMH_Enqueue Message (poly).vi"("Message"="Drag VI", "Message Queue in"=w176) -> ("error out"=w177:errorcluster)  [unwired: 8 in, 1 out]
            n212 = event-data("Discard?"=TRUE) -> ()  [unwired: 1 in, 1 out]
          }
          event "Modules Tree": Shortcut Menu Selection (User) {
            # "User selects something from the Right Click Shortcut Menu"
            n213 = event-data() -> ("ItemTag"=w180:string)  [unwired: 1 in]
            n214 = case shown="\"Open File Library on Disk\", \"Open VI on Disk\", \"Who is launching this module?\"" w180 {
              selector: w180 -> [w185 _ w191 w194 w197]
              tunnel: w181 -> [w189 _ w192 w195 w198]
              tunnel: [w190 _ w193 w196 w199] -> w182
              frame "-Run: Hide Panel", "-Run: Show Diagram", "-Run: Show Panel", "-Run: Stop Module" {
                n215 = Match Pattern(string=w185, regular expression="-Run: ") -> (after substring=w184:string)  [unwired: 1 in, 3 out]
                n216 = Bundle(cluster=T15 {"Event Name"=""} ("Execute Default Event Request Argument"), "Event Name"=w184) -> (w187:T15)
                n217 = call-poly <vilib>:"Delacor_lib_QMH_Enqueue Message (poly).vi"("Message Data"=w187, "Message"="Execute Default Event Request", "Message Queue in"=w189) -> ("error out"=w190:errorcluster)  [unwired: 7 in, 1 out]
              }
              frame Default {
              }
              frame "Open File Library on Disk", "Open VI on Disk", "Who is launching this module?" {
                n218 = call-poly <vilib>:"Delacor_lib_QMH_Enqueue Message (poly).vi"("Message"=w191, "Message Queue in"=w192) -> ("error out"=w193:errorcluster)  [unwired: 8 in, 1 out]
              }
              frame "Who is registered to this module's broadcasts?" {
                n219 = call-poly <vilib>:"Delacor_lib_QMH_Enqueue Message (poly).vi"("Message"=w194, "Message Queue in"=w195) -> ("error out"=w196:errorcluster)  [unwired: 8 in, 1 out]
              }
              frame "Open Module API Tester", "Search for Event Callers / listeners" {
                n220 = call-poly <vilib>:"Delacor_lib_QMH_Enqueue Message (poly).vi"("Message"=w197, "Message Queue in"=w198) -> ("error out"=w199:errorcluster)  [unwired: 8 in, 1 out]
              }
            }
          }
          event "Modules Tree": Value Change {
            w202 = TRUE  # Tree valid Selection
            # "The user selected an item on the tree control"
            n221 = event-data() -> ()  [unwired: 1 in, 1 out]
            n222 = Bundle(cluster=T16 {"Tree DQMH Sel"=""} ("Tree DQMH Selection Argument"), "Tree DQMH Sel"="Modules Tree") -> (w203:T16)
            n223 = call "Validate if event is selected.vi"("Tree Selection"="Modules Tree") -> ("Selection type"=w200:T4)  [unwired: 10 in]
            n224 = call-poly <vilib>:"Delacor_lib_QMH_Enqueue Message (poly).vi"("Message Data"=w203, "Message"="Tree DQMH Selection", "Message Queue in"=w206) -> ("error out"=w207:errorcluster)  [unwired: 7 in, 1 out]
          }
          event "Modules Tree": Shortcut Menu Activation? {
            # "This is wher the shorcut menu is filled, only after the user select a module"
            n225 = event-data() -> ("MenuRef"=w211:refnum<k9>)  [unwired: 1 in]
            n226 = call "Create Tree Shortcut Menu.vi"("Selection type"=w210, "Menu in"=w211) -> ("error out"=w212:errorcluster)  [unwired: 9 in]
            n227 = Not(x=w208) -> (.not. x?=w209:bool)
            n228 = event-data("Discard?"=w209) -> ()  [unwired: 1 in, 1 out]
          }
          event "Projects": Value Change {
            n229 = event-data() -> ()  [unwired: 1 in, 1 out]
            n230 = call-poly <vilib>:"Delacor_lib_QMH_Enqueue Message (poly).vi"("Message Data"="Projects", "Message"="Refresh Targets", "Message Queue in"=w215) -> ("error out"=w216:errorcluster)  [unwired: 7 in, 1 out]
          }
          event "Projects": Shortcut Menu Activation? {
            n231 = event-data() -> ("MenuRef"=w225:refnum<k9>)  [unwired: 1 in]
            n232 = Delete Menu Items(9:w225) -> (0:w223:errorcluster, 3:w224:refnum<k9>)  [unwired: 3 in]
            n233 = Insert Menu Items(6:w223, 8:string[] ["Open Project Folder", "Edit Project Description", "Open Antidoc Output"] ("item names"), 9:w224) -> (0:w219:errorcluster)  [unwired: 3 in, 2 out]
            n234 = local read "Projects"() -> (w221:string)
            n235 = Empty String/Path?(string/path=w221) -> (empty?=w220:bool)
            n236 = event-data("Discard?"=w220) -> ()  [unwired: 1 in, 1 out]
          }
          event "Projects": Shortcut Menu Selection (User) {
            n237 = event-data() -> ("ItemTag"=w228:string)  [unwired: 1 in]
            n238 = call-poly <vilib>:"Delacor_lib_QMH_Enqueue Message (poly).vi"("Message"=w228, "Message Queue in"=w229) -> ("error out"=w230:errorcluster)  [unwired: 8 in, 1 out]
          }
          event "Theme": Value Change {
            # "#via_ignore Wired Terminals in Subdiagrams"
            # "Another Module called the \"Scan DQMH Modules\" API Method."
            n239 = event-data() -> ()  [unwired: 1 in, 1 out]
            n240 = call-poly <vilib>:"Delacor_lib_QMH_Enqueue Message (poly).vi"("Message Data"="Theme", "Message"="Theme", "Message Queue in"=w237) -> ("error out"=w238:errorcluster)  [unwired: 7 in, 1 out]
          }
          event User Event {
            # "Another Module called the \"Expand or Close\" API Method."
            n241 = event-data() -> ("Expand?"=w241:bool)  [unwired: 1 in]
            n242 = Bundle(cluster=T14 {"Expand?"=FALSE} ("Expand or Close Argument"), "Expand?"=w241) -> (w242:T14)
            n243 = call-poly <vilib>:"Delacor_lib_QMH_Enqueue Message (poly).vi"("Message Data"=w242, "Message"="Expand or Close", "Message Queue in"=w245) -> ("error out"=w246:errorcluster)  [unwired: 7 in, 1 out]
          }
          event User Event {
            # "Another Module called the \"Get Module Execution Status\" API Method."
            n244 = event-data() -> ()  [unwired: 1 in, 1 out]
            n245 = call "Update Module Execution Status.vi"("Running?"=TRUE) -> ("error out"=w250:errorcluster)  [unwired: 10 in]
          }
          event User Event {
            # "Hide the panel of this VI, and send a status updated message to let listeners know."
            # "Another Module called the \"Hide Panel\" API Method."
            n246 = event-data() -> ()  [unwired: 1 in, 1 out]
            n247 = control-ref of="This VI"() -> (w253:refnum<vi>)
            n248 = call "Hide VI Panel.vi"("VI"=w253) -> ()  [unwired: 10 in, 1 out]
          }
          event User Event {
            # "Another Module called the \"Scan DQMH Modules\" API Method."
            n249 = event-data() -> ("Include Dependencies"=w258:bool, "Project"=w257:string, "Target"=w254:string)  [unwired: 1 in]
            n250 = Bundle(cluster=T17 {"Include Dependencies"=FALSE, "Project"="", "Target"=""} ("Scan DQMH Modules Argument"), "Include Dependencies"=w258, "Project"=w257, "Target"=w254) -> (w259:T17)
            n251 = call-poly <vilib>:"Delacor_lib_QMH_Enqueue Message (poly).vi"("Message Data"=w259, "Message"="Scan DQMH Modules", "Message Queue in"=w262) -> ("error out"=w263:errorcluster)  [unwired: 7 in, 1 out]
          }
          event Value Change {
            # "#via_ignore Unwired Event Nodes"
            # "Another Module called the \"Scan DQMH Modules\" API Method."
            n252 = event-data() -> ()  [unwired: 1 in, 1 out]
            n253 = local read "Projects"() -> (w267:string)
            n254 = Empty String/Path?(string/path="Targets") -> (empty?=w264:bool)
            n255 = Empty String/Path?(string/path=w267) -> (empty?=w270:bool)
            n256 = Or(x=w270, y=w264) -> (x .or. y?=w265:bool)
            n257 = case shown="False" w265 {
              tunnel: [w280 _] -> w272
              tunnel: w271 -> [w279 _]
              tunnel: w267 -> [w274 _]
              tunnel: "Targets" -> [w273 _]
              frame False {
                n258 = Bundle(cluster=T17 {"Include Dependencies"=FALSE, "Project"="", "Target"=""} ("Scan DQMH Modules Argument"), "Include Dependencies"="Include Dependencies", "Project"=w274, "Target"=w273) -> (w276:T17)
                n259 = call-poly <vilib>:"Delacor_lib_QMH_Enqueue Message (poly).vi"("Message Data"=w276, "Message"="Scan DQMH Modules", "Message Queue in"=w279) -> ("error out"=w280:errorcluster)  [unwired: 7 in, 1 out]
              }
              frame True {
                n260 = call "Status Updated.vi"("Status"=" To Scan, Please, first Select a Project and a target") -> ()  [unwired: 10 in, 1 out]
              }
            }
          }
          event User Event {
            # "Another Module called the \"Show Diagram\" API Method. This event is used for debugging."
            n261 = event-data() -> ()  [unwired: 1 in, 1 out]
            n262 = disable-structure shown="RUN_TIME_ENGINE==False" {
              disable-tunnel: w282 -> [w285 _]
              frame condition #0 (active) {
                # "functionality not available in exe"
                n263 = invoke on="Invoke Node" class="VI" method="Lock State.Get"() -> (error out=w291:errorcluster, "Get Lock State"=w290:T18, "pwd in cache"=w287:bool)  [unwired: 4 in, 1 out]
                n264 = Equal?(x=T18."Password-protected", y=w290) -> (x = y?=w288:bool)
                n265 = Compound Arithmetic op=AND(w288, invert w287) -> (w286:bool)
                n266 = case shown="False" w286 {
                  tunnel: w291 -> [w294 _]
                  tunnel: w285 -> [w292 _]
                  frame False {
                    n267 = case shown="False" w292 {
                      frame False {
                      }
                      frame True {
                      }
                    }
                    n268 = property on="Property Node" class="VI"(error in=w294, "BDWin.Open"=TRUE ("Block Diagram Window:Open")) -> ()  [unwired: 1 in, 2 out]
                  }
                  frame True {
                    # "Password-protected VI, and the password is not in the cache. Do not show the diagram."
                  }
                }
              }
              frame condition #1 {
              }
            }
          }
          event User Event {
            # "Show the panel of this VI, and send a status updated message to let listeners know."
            # "Another Module called the \"Show Panel\" API Method."
            n269 = event-data() -> ()  [unwired: 1 in, 1 out]
            n270 = disable-structure shown="Default" {
              disable-tunnel: w295 -> [w298 _]
              frame condition #0 (active) {
                n271 = control-ref of="This VI"() -> (w299:refnum<vi>)
                n272 = call "Open VI Panel.vi"("VI"=w299) -> ()  [unwired: 10 in, 1 out]
                n273 = case shown="True" w298 {
                  frame False {
                  }
                  frame True {
                  }
                }
              }
              frame condition #1 {
                # "Scripting not\nallowed on RTE\nIn case someone left Panther Dashboard\nunder dependencies."
              }
            }
          }
          event User Event {
            # "The Stop Module Event can get fired from the Exit message in the MHL. The queue gets destroyed in that case. If the queue no longer exists, the Enqueue Exit as a priority message will return error 1. It is safe to ignore, because the module is already exiting."
            # "Another Module called the \"Stop Module\" API Method  or the Message Handling Loop below."
            n274 = event-data() -> ("Origin"=w308:string, "Exit via Stop Module Req?"=w304:bool, "Wait for Module to stop?"=w303:bool)  [unwired: 1 in]
            n275 = local write "Messages"(w308) -> ()
            n276 = Bundle By Name(cluster=T19 {"Origin"="", "Exit via Stop Module Req?"=FALSE, "Wait for Module to stop?"=FALSE} ("Stop Argument"), "Exit via Stop Module Req?"=w304, "Wait for Module to stop?"=w303) -> (w302:T19)
            n277 = call-poly <vilib>:"Delacor_lib_QMH_Enqueue Message (poly).vi"("Priority Message? (F)"=TRUE, "Message Data"=w302, "Message"="Exit", "Message Queue in"=w309) -> ("error out"=w313:errorcluster)  [unwired: 6 in, 1 out]
            n278 = call <vilib>:"Clear Errors.vi"("error in (no error)"=w313, "specific error code to clear (0: all)"=1) -> ("error out"=w312:errorcluster)  [unwired: 4 in, 1 out]
          }
          event Panel Close? {
            w319 = TRUE  # Discard the event, the MHL is responsible for closing and stopping this VI.
            # "Hide the panel or send the 'Exit' message if the user clicks the 'X' on the module main VI panel."
            n279 = event-data() -> ()  [unwired: 1 in, 1 out]
            n280 = call-poly <vilib>:"Delacor_lib_QMH_Enqueue Message (poly).vi"("Priority Message? (F)"=TRUE, "Message"="Exit", "Message Queue in"=w318) -> ("error out"=w320:errorcluster)  [unwired: 7 in, 1 out]
            n281 = event-data ("Event Filter Node")("Discard?"=w319) -> ()  [unwired: 1 in, 1 out]
          }
          event Timeout {
            n282 = event-data() -> ()  [unwired: 1 in, 1 out]
            n283 = call "Scan For App Projects.vi"() -> ("error out"=w323:errorcluster)  [unwired: 11 in]
          }
        }
        n284 = call-dynamic "Delacor_lib_QMH_Error Handler - Event Handling Loop.vi"("error in"=w92, "Message Queue in"=w87) -> ("dup error in"=w91:errorcluster)  [unwired: 8 in, 1 out]
      }
      n285 = while {
        tunnel: w29 -> [w46]
        tunnel: [w45] -> w28
        shift-right: [w43] -> _
        shift-left: -1 -> [w42]
        shift-right: [w41] -> _
        shift-left: _ -> [w40]
        tunnel: w26 -> [w39]
        tunnel: [w47] -> w33
        shift-right: [w38] -> _
        shift-left: _ -> [w37]
        stop <- w44 stop-if-true
        # "Helper Loop"
        n286 = event shown="[4] <Panther Dashboard Broadcast Events.Targets Updated>: User Event" {
          selector: w46 -> [_ _ _ _ _ _]
          dyn-events: [_ _ _ _ _ _] -> w45
          timeout: w42 -> [_ _ _ _ _ _]
          tunnel: [_ TRUE _ _ _ _] -> w44
          tunnel: [w50 w55 w60 w71 w76 w79] -> w41
          tunnel: [w51 w56 500 w70 w75 w78] -> w43
          tunnel: w42 -> [w51 w56 _ w70 w75 w78]
          tunnel: w40 -> [w50 w55 _ w71 w76 w79]
          tunnel: [w52 _ _ _ _ _] -> w48
          tunnel: [w49 w53 w58 w69 w73 w77] -> w38
          tunnel: w37 -> [w49 w53 _ w69 w73 w77]
          event Timeout {
            n287 = event-data() -> ()  [unwired: 1 in, 1 out]
            n288 = call "Get Module Execution Status by ref.vi"("Modules Tree ref"=w49, "Refs"=w50) -> ("error out"=w52:errorcluster)  [unwired: 9 in]
          }
          event User Event {
            n289 = event-data() -> ()  [unwired: 1 in, 1 out]
            n290 = Unbundle By Name(w55) -> ("Modules"=w54:refnum<vi>[])
            n291 = Close Reference(reference=w54) -> ()  [unwired: 1 in, 1 out]
          }
          event User Event {
            # "Refresh time"
            n292 = event-data() -> ("Modules"=w63:refnum<vi>[], "Modules Types"=w61:T9[], "Application Instance"=w62:refnum<vi>)  [unwired: 1 in]
            n293 = Bundle By Name(cluster=T11 {"Modules"=[], "Modules Types"=[], "Application Instance"=refnum}, "Modules"=w63, "Modules Types"=w61, "Application Instance"=w62) -> (w60:T11)
            n294 = control-ref of="Modules Tree"() -> (w59:refnum<vi>)
            n295 = call "Set Tree custom symbols.vi"("TreeControl in"=w59) -> ("TreeControl out"=w58:refnum<vi>)  [unwired: 10 in]
          }
          event User Event {
            n296 = event-data() -> ("Projects"=w68:string[])  [unwired: 1 in]
            n297 = control-ref of="Projects"() -> (w67:refnum<vi>)
            n298 = Index Array(array=w68) -> (element=w66:string)  [unwired: 1 in]
            n299 = property class="CmbBox"(reference=w67, "Strings[]"=w68, "Val(Sgnl)"=w66) -> ()  [unwired: 1 in, 2 out]
          }
          event User Event {
            n300 = event-data() -> ("Targets"=w72:string[])  [unwired: 1 in]
            n301 = control-ref of="Targets"() -> (w74:refnum<vi>)
            n302 = property class="CmbBox"(reference=w74, "Strings[]"=w72) -> ()  [unwired: 1 in, 2 out]
          }
          event User Event {
            n303 = event-data() -> ("Status"=→"Messages":string)  [unwired: 1 in]
          }
        }
        n304 = call-dynamic "Delacor_lib_QMH_Error Handler - Helper Loop.vi"("error in"=w48, "Message Queue in"=w39) -> ("dup error in"=w47:errorcluster)  [unwired: 8 in, 1 out]
      }
    }
    frame Error {
      # "Synchronize Caller Events.vi will inform Start Module.vi that the module has launched and will let the code calling Start Module.vi register for broadcasts and would permit the caller receive the broadcast that an error occurred at launch time."
      n305 = call-dynamic "Delacor_lib_QMH_Release Message Queue.vi"("error in"=w689, "Message Queue"=w682) -> ("error out"=w688:errorcluster)  [unwired: 9 in]
      n306 = call "Synchronize Caller Events.vi"("Singleton Module Admin in"=w683) -> ("error out"=w690:errorcluster)  [unwired: 9 in, 1 out]
      n307 = call "Module Name--constant.vi"() -> ("Module Name"=w686:string)  [unwired: 11 in]
      n308 = Format Into String(format string="An error occurred during initialization. %s is no longer running.", w686) -> (resulting string=w684:string)  [unwired: 2 in, 1 out]
      n309 = Merge Errors(w688, w690) -> (w691:errorcluster)
      n310 = call "Error Reported.vi"("Additional Information"=w684, "Error"=w691) -> ()  [unwired: 9 in, 1 out]
    }
  }
  n311 = Merge Errors(w18, w21, w12) -> (w17:errorcluster)
  n312 = call "Close Module.vi"("error in (no error)"=w17, "Module Admin in"=w11) -> ("error out"=w19:errorcluster, "External Launch"=w5:bool, "Module Admin out"=w6:refnum<class "Delacor_lib_QMH_Module Admin.lvclass">)  [unwired: 7 in]
  n313 = Unregister For Events(event registration refnum=w3) -> ()  [unwired: 1 in, 1 out]
  n314 = Unregister For Events(event registration refnum=w10, error in=w19) -> (error out=w16:errorcluster)
  "error out" <- w16
  n315 = case "External Launch?" shown="True" w5 {
    tunnel: w16 -> [_ w692]
    frame False {
    }
    frame True {
      n316 = case shown="No Error" w692 {
        frame No Error {
          n317 = invoke class="VI" method="FP.Close"() -> ()  [unwired: 3 in, 3 out]
        }
        frame Error {
          n318 = invoke on="Invoke Node" class="VI" method="FP.Open"("Activate"=TRUE ("Activate?")) -> ()  [unwired: 4 in, 5 out]
        }
      }
    }
  }
  n319 = local write "Module Admin"(w6) -> ()
